vi "from string.vi"(8 "error in":errorcluster, 9 "data":string, 10 "version":string, 11 "fixed channel configuration in":refnum<class "ActiveFrontEndModule configuration.lvclass">) -> (0 "error out":errorcluster, 3 "fixed channel configuration out":refnum<class "ActiveFrontEndModule configuration.lvclass">)   [LabVIEW 2017, in "ActiveFrontEndModule configuration.lvclass"]
doc: "Provides an interface for loading a module configuration from a file or other serialized data source. It is recommended that all children of this class store data in two sets--data required for its own initialization, and any data required for parent initialization--and that each implementation uses the <b>Call Parent Method</b> primitive to de-serialize parent information. As a result, it is expected that every module configuration class calls <b>component configuration.lvclass:From String.vi</b>.\nNI Tag Bus Module Framework 1.0.3.43\nNI Systems Engineering"
uses:
  ActiveFrontEndModule configuration.lvclass
  ActiveFrontEndModule configuration.lvclass/ActiveFrontEndModule configuration.ctl
  <vilib>/NI/JSON Support for LabVIEW/JSON Data Classes/JSON Helper/Parsing/Parse Value.vi
  <vilib>/NI/JSON Support for LabVIEW/JSON Data Classes/JSON Helper/To More Specific Type (Object).vi
  <vilib>/NI/JSON Support for LabVIEW/JSON Data Classes/JSON Object/Get Parameter Value.vi
  <vilib>/NI/JSON Support for LabVIEW/JSON Data Classes/JSON Object/Get Value (JSON).vi
  <vilib>/NI/JSON Support for LabVIEW/JSON Data Classes/JSON Datatype/JSON Null.lvclass
  <vilib>/NI/JSON Support for LabVIEW/JSON Data Classes/JSON Object/Get Parameter XNode/Get Object Parameters.xnode
  <vilib>/NI/JSON Support for LabVIEW/JSON Data Classes/JSON Object/JSON Object.lvclass
  <vilib>/NI/DCAF/Tag Editor Core/control module/configuration/control module configuration.lvclass
  <vilib>/NI/Configuration Framework/serializable configuration/NISE_CEF_serializable configuration.lvclass
  <vilib>/NI/JSON Support for LabVIEW/JSON Data Classes/JSON Helper/JSON Helper.lvclass
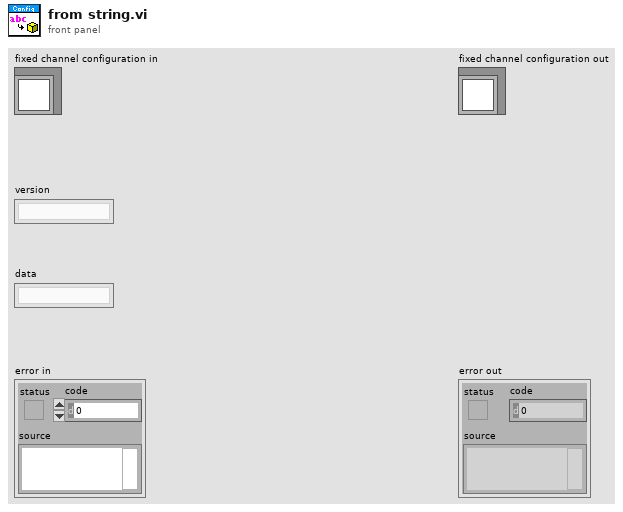
[diagram p1: front panel]
types:
  T1 = typedef "ActiveFrontEnd.lvlib/Parameters.ctl" = cluster{"VDCLink_setpt":sgl, "VDCLinkRampRate":sgl, "Q_setpt":sgl, "Pf_setpt":sgl, "Mode":T2, "perturbance_amp":sgl, "perturbance_freq":sgl, "dT":sgl}
  T2 = typedef "ActiveFrontEnd.lvlib/Mode.ctl" = enum16{"Q Control", "Pf Control"}
  T3 = typedef "ActiveFrontEnd.lvlib/PI_Settings.ctl" = cluster{"gains":T4, "output range":T5, "PI_state":enum8{"idle", "normal", "manual", "perturbance"}, "reset":bool, "manual":sgl}
  T4 = typedef "niFpgaPID_PIGains.ctl" = cluster{"proportional gain":sgl, "integral gain":sgl}
  T5 = typedef "niFpgaPID_OutputRange.ctl" = cluster{"output high (Inf)":sgl, "output low (-Inf)":sgl}
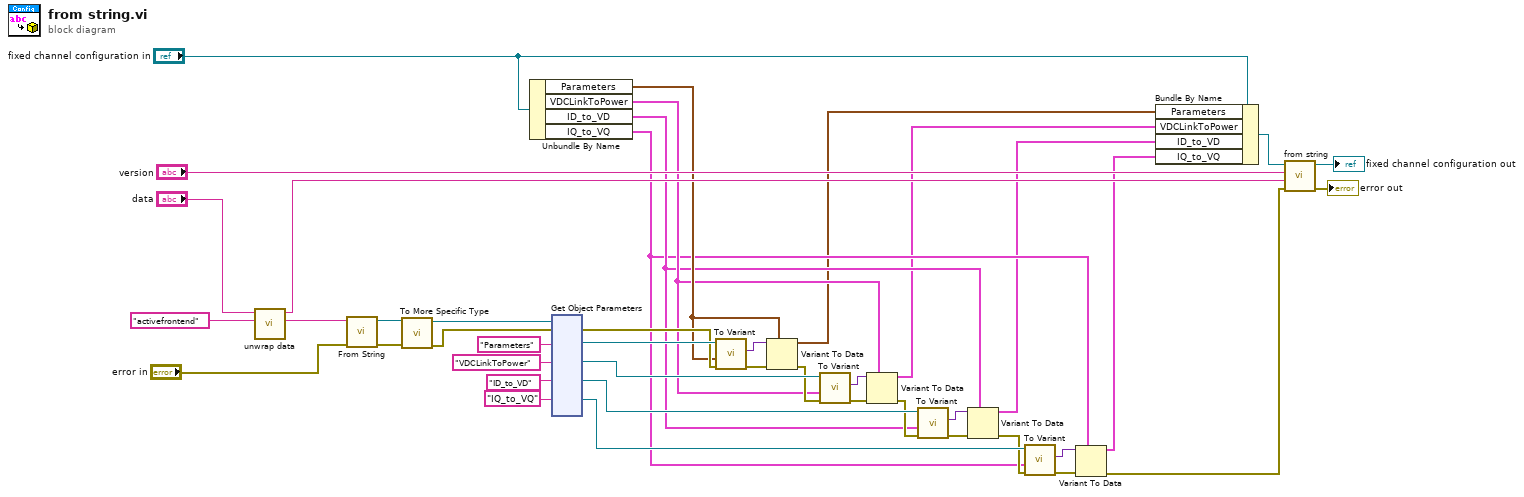
[diagram p0: block diagram]
diagram:
  n1 = call <vilib>:"unwrap data.vi"("identifier"="activefrontend", "data to unwrap"="data") -> ("unwrapped data"=w37:string, "remaining string"=w38:string)  [unwired: 8 in]
  n2 = call <vilib>:"From String.vi"("error in (no error)"="error in", "JSON String"=w37) -> ("error out"=w35:errorcluster, "JSON out"=w34:refnum<class "JSON Null.lvclass">)  [unwired: 8 in]
  n3 = call-poly <vilib>:"To More Specific Type.vi"("error in (no error)"=w35, "JSON Datatype in"=w34) -> ("error out"=w32:errorcluster, "JSON Datatype out"=w33:refnum<class "JSON Object.lvclass">)  [unwired: 8 in]
  n4 = Unbundle By Name("fixed channel configuration in") -> ("Parameters"=w21:T1, "VDCLinkToPower"=w16:T3, "ID_to_VD"=w12:T3, "IQ_to_VQ"=w8:T3)
  n5 = xnode "Get Object Parameters"("key"="Parameters", "key"="VDCLinkToPower", "key"="ID_to_VD", "key"="IQ_to_VQ", "JSON Object In"=w33, "error in"=w32) -> ("parameter"=w27:refnum<class "JSON Null.lvclass">, "parameter"=w26:refnum<class "JSON Null.lvclass">, "parameter"=w25:refnum<class "JSON Null.lvclass">, "parameter"=w24:refnum<class "JSON Null.lvclass">, "error out"=w23:errorcluster)
  n6 = call <vilib>:"To Variant.vi"("error in (no error)"=w23, "datatype and defaults"=w21, "JSON Datatype in"=w27) -> ("error out"=w22:errorcluster, "Variant"=w20:variant)  [unwired: 6 in, 1 out]
  n7 = Variant To Data(error in=w22, type=w21, Variant=w20) -> (data=w5:T1, error out=w19:errorcluster)
  n8 = call <vilib>:"To Variant.vi"("error in (no error)"=w19, "datatype and defaults"=w16, "JSON Datatype in"=w26) -> ("error out"=w18:errorcluster, "Variant"=w17:variant)  [unwired: 6 in, 1 out]
  n9 = Variant To Data(error in=w18, type=w16, Variant=w17) -> (data=w4:T3, error out=w15:errorcluster)
  n10 = call <vilib>:"To Variant.vi"("error in (no error)"=w15, "datatype and defaults"=w12, "JSON Datatype in"=w25) -> ("error out"=w14:errorcluster, "Variant"=w13:variant)  [unwired: 6 in, 1 out]
  n11 = Variant To Data(error in=w14, type=w12, Variant=w13) -> (data=w3:T3, error out=w11:errorcluster)
  n12 = call <vilib>:"To Variant.vi"("error in (no error)"=w11, "datatype and defaults"=w8, "JSON Datatype in"=w24) -> ("error out"=w10:errorcluster, "Variant"=w9:variant)  [unwired: 6 in, 1 out]
  n13 = Variant To Data(error in=w10, type=w8, Variant=w9) -> (data=w2:T3, error out=w1:errorcluster)
  n14 = Bundle By Name(cluster="fixed channel configuration in", "Parameters"=w5, "VDCLinkToPower"=w4, "ID_to_VD"=w3, "IQ_to_VQ"=w2) -> (w6:refnum<class "ActiveFrontEndModule configuration.lvclass">)
  n15 = call-parent <vilib>:"from string.vi"("error in"=w1, "data"=w38, "version"="version", "fixed channel configuration in"=w6) -> ("error out"=→"error out":errorcluster, "fixed channel configuration out"=→"fixed channel configuration out":refnum<class "ActiveFrontEndModule configuration.lvclass">)  [unwired: 6 in]
